vi "Close Web Service.vi"(8 "error in (no error)":errorcluster, 11 "ContactAndRegisterWithNmaSapService refnum":refnum<k24>) -> (0 "error out":errorcluster)   [LabVIEW 2023, in "ContactAndRegisterWithNmaSapService.lvlib"]
uses:
  <userlib>/WebService/_ContactAndRegisterWithNmaSapService/ContactAndRegisterWithNmaSapService.dll
  <userlib>/WebService/_ContactAndRegisterWithNmaSapService/ContactAndRegisterWithNmaSapService.lvlib
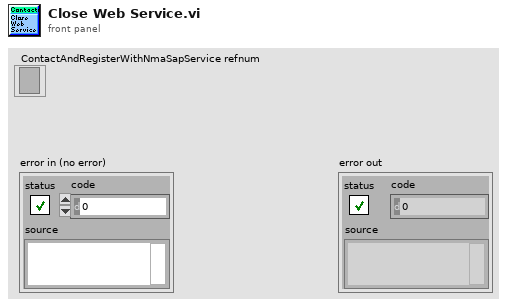
[diagram p1: front panel]
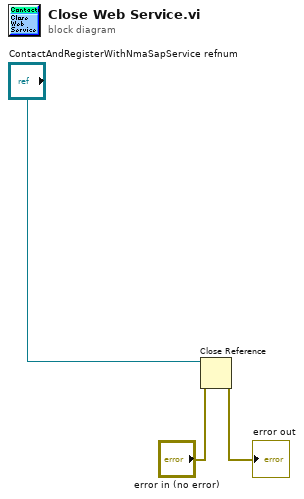
[diagram p0: block diagram]
diagram:
  n1 = Close Reference(reference="ContactAndRegisterWithNmaSapService refnum", error in (no error)="error in (no error)") -> (error out=→"error out":errorcluster)
